vi "True Straight - Arcade T Test.vi"(0 "Fwd/Rev Joy":dbl step=0.1, 7 "Bypass":bool, 11 "Left/Right Joy":dbl step=0.1, 12 "Left Encoder":dbl step=0.1, 14 "Right Encoder":dbl step=0.1) -> (4 "Fwd/Rev Out":dbl, 10 "Left/Right Out":dbl, 15 "Encoder Reset":bool)   [LabVIEW 2015]
uses:
  <vilib>/functionblocks/Edge Detection/One Shot Rising with Input/One Shot Rising with Input.vi
  <vilib>/functionblocks/FB Core/FB Core.xnode
  <vilib>/functionblocks/NI_FunctionBlock Libraries.lvlib
panel:
  out "Left/Right Bypass":bool
  out "Fwd/Rev Bypass":bool
  out "Difference":dbl
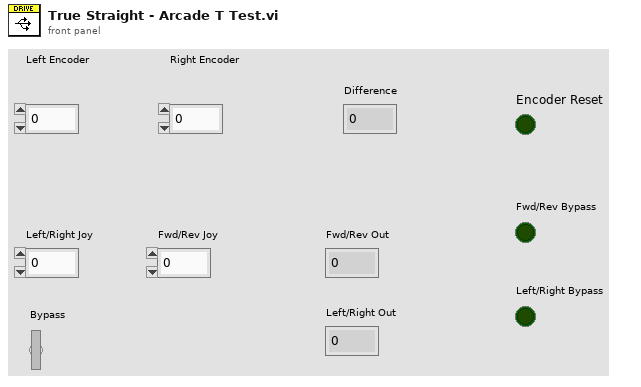
[diagram p1: front panel]
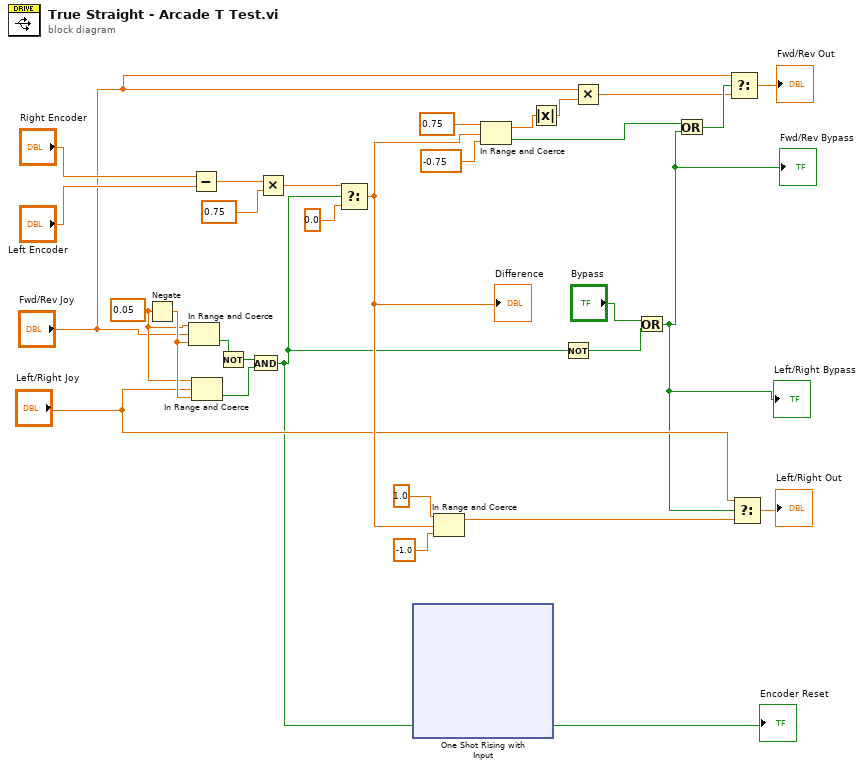
[diagram p0: block diagram]
diagram:
  w11 = 0.05
  n1 = Negate(x=w11) -> (-x=w12:dbl)
  n2 = In Range and Coerce(upper limit=w11, x="Fwd/Rev Joy", lower limit=w12) -> (In Range?=w9:bool)  [unwired: 1 out]
  n3 = Subtract(x="Right Encoder", y="Left Encoder") -> (x-y=w31:dbl)
  n4 = In Range and Coerce(upper limit=w11, x="Left/Right Joy", lower limit=w12) -> (In Range?=w8:bool)  [unwired: 1 out]
  n5 = Not(x=w9) -> (.not. x?=w10:bool)
  n6 = And(x=w10, y=w8) -> (x .and. y?=w3:bool)
  n7 = Multiply(x=w31, y=0.75) -> (x*y=w29:dbl)
  n8 = Select(t=w29, s=w3, f=0.0) -> (s? t:f=w16:dbl)
  "Difference" <- w16
  n9 = xnode "One Shot Rising with Input"("input"=w3) -> ("output"=→"Encoder Reset":bool)  [unwired: 1 in, 1 out]
  n10 = In Range and Coerce(upper limit=1.0, x=w16, lower limit=-1.0) -> (coerced(x)=w27:dbl)  [unwired: 1 out]
  n11 = In Range and Coerce(upper limit=0.75, x=w16, lower limit=-0.75) -> (coerced(x)=w13:dbl, In Range?=w19:bool)
  n12 = Absolute Value(x=w13) -> (abs(x)=w14:dbl)
  n13 = Not(x=w3) -> (.not. x?=w4:bool)
  n14 = Multiply(x="Fwd/Rev Joy", y=w14) -> (x*y=w15:dbl)
  n15 = Or(x="Bypass", y=w4) -> (x .or. y?=w1:bool)
  "Fwd/Rev Bypass" <- w1
  "Left/Right Bypass" <- w1
  n16 = Or(x=w19, y=w1) -> (x .or. y?=w20:bool)
  n17 = Select(t="Fwd/Rev Joy", s=w20, f=w15) -> (s? t:f=→"Fwd/Rev Out":dbl)
  n18 = Select(t="Left/Right Joy", s=w1, f=w27) -> (s? t:f=→"Left/Right Out":dbl)
